vi "novoGoleiroAlinharComATrave.vi"(8 "balls":T1[](array[typedef]), 9 "Robot in":T2, 10 "Goleiro.X_padrao":dbl, 11 "IA State":T7={"our_robots"=[], "enemy_robots"=[], "balls"=[], "geometry"={"field_length"=0, "field_width"=0, "goal_width"=0, "goal_depth"=0, "center_circle_radius"=0, "defense_width"=0, "defense_depth"=0, "free_kick_from_defense_dist"=0, "penalty_spot_from_field_line_dist"=0, "penalty_line_from_spot_dist"=0, "half_moon_depth"=0, "half_moon_width"=0}, "IA Judge"={"stage"="", "command"="", "our_goalie_id"=0.0, "enemy_goalie_id"=0.0, "command enum"=enum."Halt", "Time"=enum."Azul"}, "Received Timestamp"=timestamp(0 s since 1904-01-01), "Events"={"Touch"=FALSE, "id touch"=0.0, "Ball out of \nVision"=FALSE, "Ball inside \nGoalie area"=FALSE, "Robot not responding"=FALSE, "Robots responding status"=[1.0, 1.0, 1.0, 1.0, 1.0, 1.0], "Enemy Ball \nPossession"=FALSE, "Id ini Possession"=0.0, "Ball Possesion"=FALSE, "Id Possesion"=0.0, "Ball at\nour goal side"=FALSE, "Ball at\ntouchline"=FALSE, "Ball at\nenemy goal side"=FALSE}}) -> (3 "Cluster de saída":T2)   [LabVIEW 2018]
uses:
  2019/VSS/Core/AI Input.ctl
  2019/VSS/Core/AI Robot.ctl
  2019/VSS/Intel/Functions Enum.ctl
  2019/VSS/Intel/AttackerStates.ctl
  2019/VSS/Path Planning/RRT/PathDests.ctl
  2019/VSS/Path Planning/RRT/PathDest.ctl
  2019/VSS/Core/AI Ball.ctl
  2019/VSS/Core/Field Size.ctl
  2019/VSS/Core/AI Judge.ctl
  2019/VSS/Intel/Command Enum.ctl
  2019/VSS/Util/Events/Events.ctl
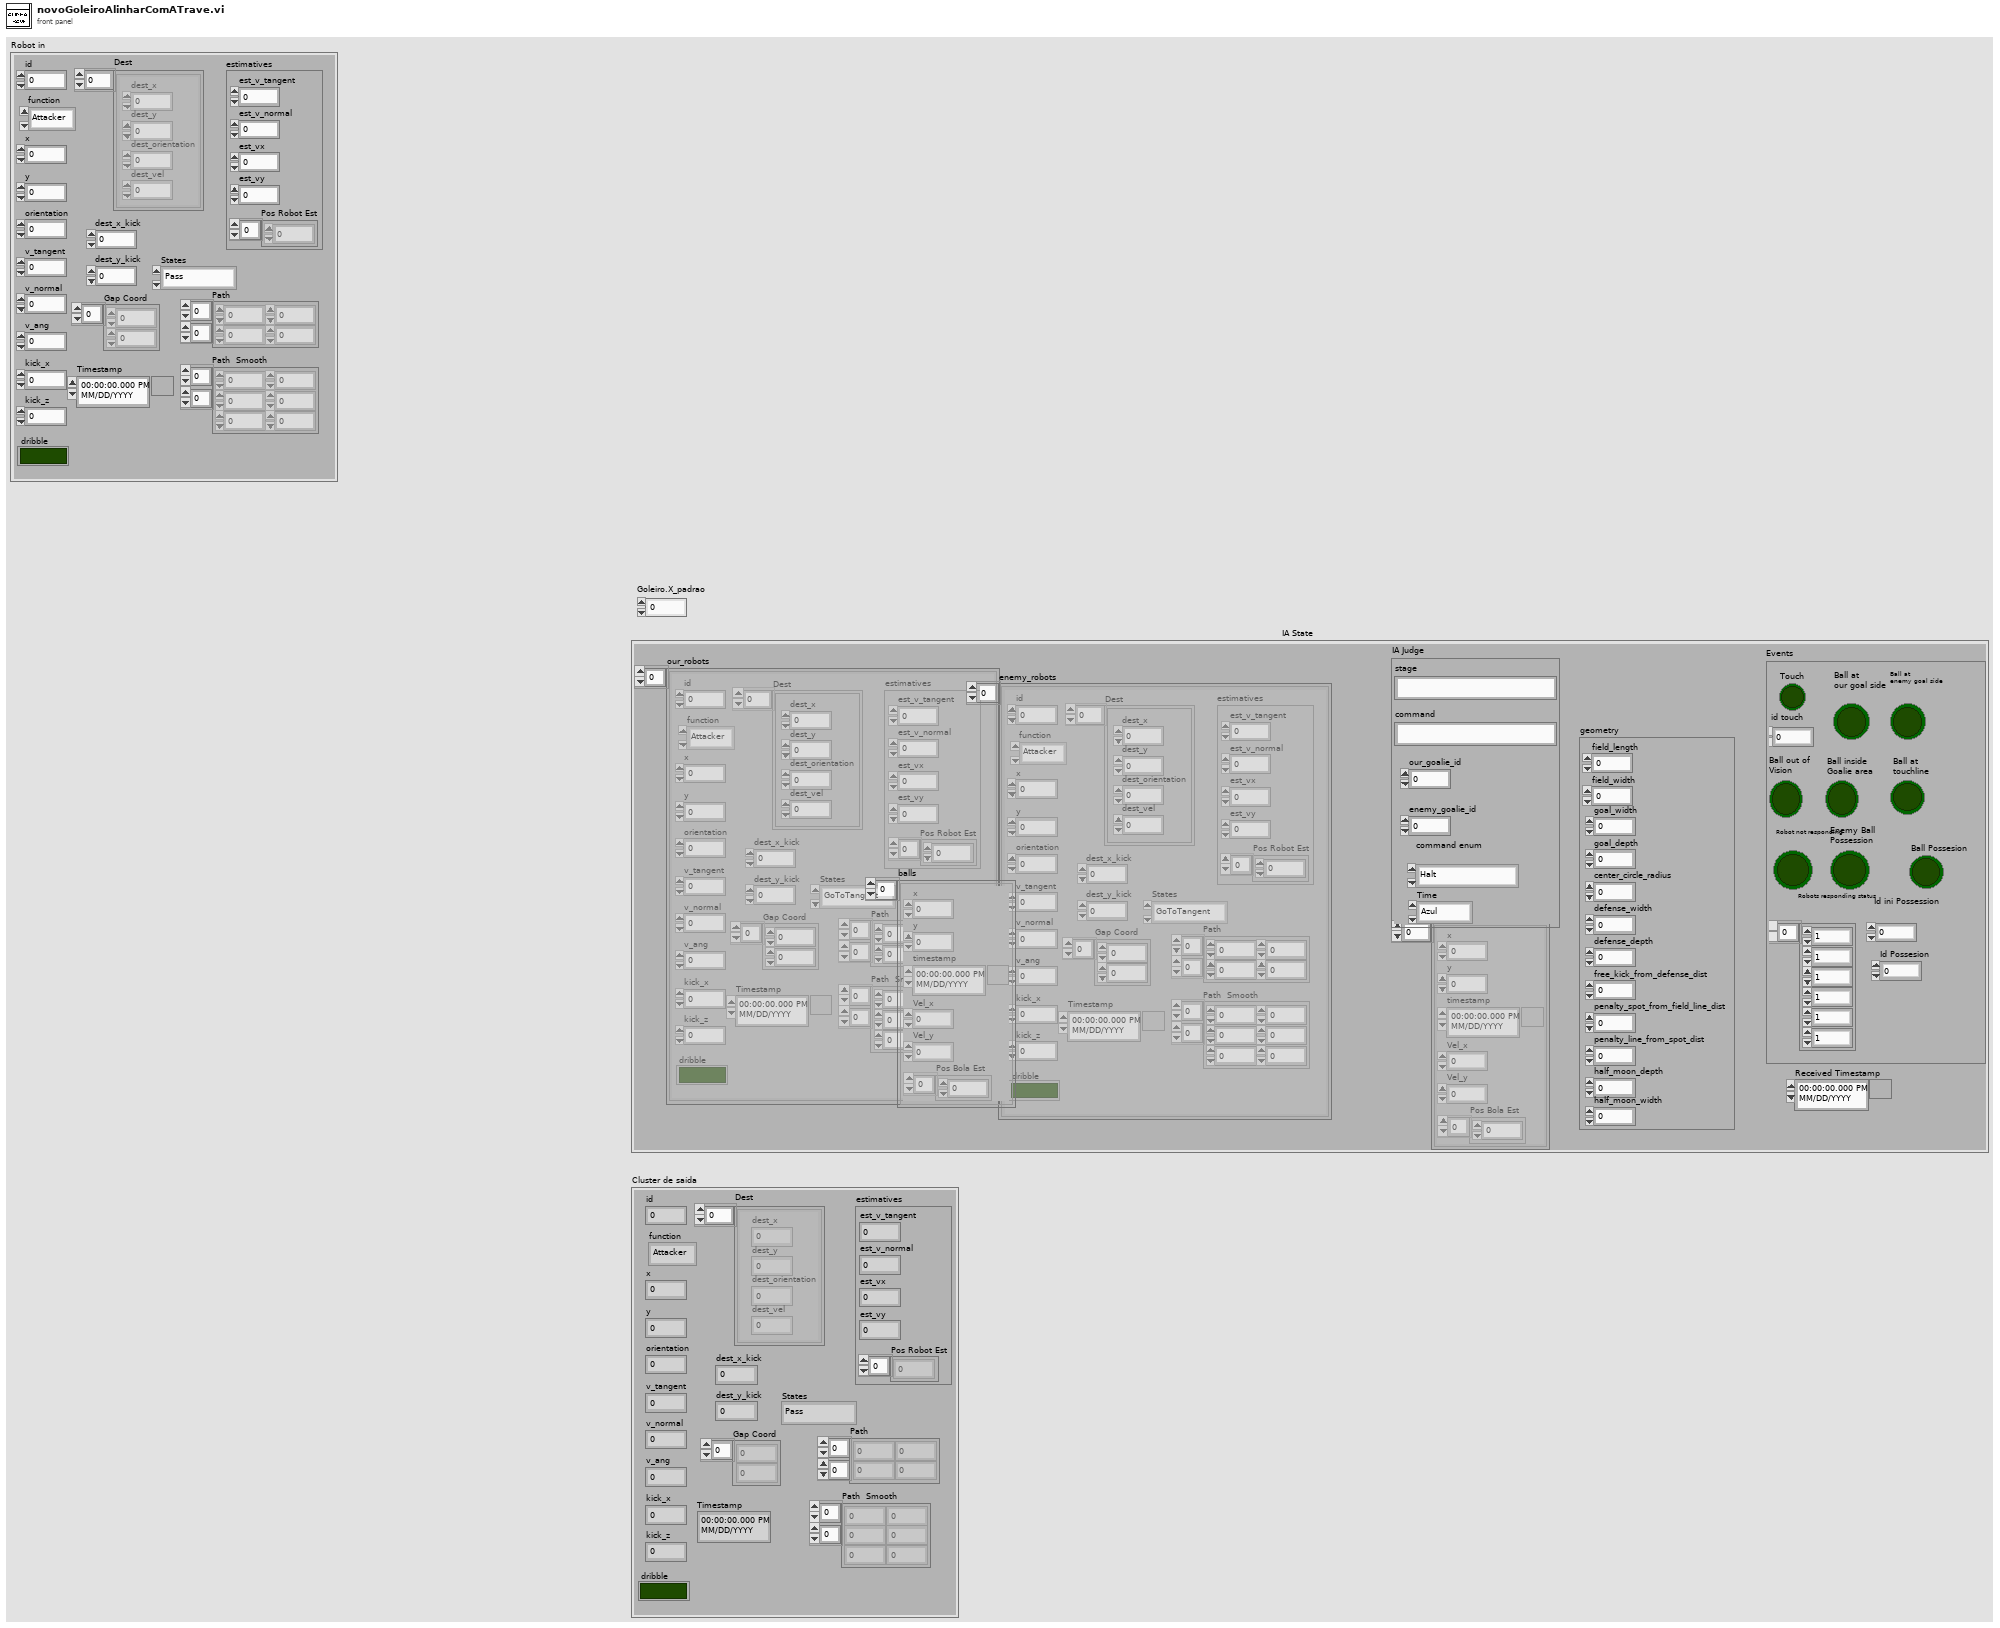
[diagram p1: front panel]
types:
  T1 = typedef "AI Ball.ctl" = cluster{"x":dbl, "y":dbl, "timestamp":timestamp, "Vel_x":dbl, "Vel_y":dbl, "Pos Bola Est":dbl[]}
  T2 = typedef "AI Robot.ctl" = cluster{"id":u32, "function":T3, "x":dbl, "y":dbl, "orientation":dbl, "v_tangent":dbl, "v_normal":dbl, "v_ang":dbl, "kick_x":dbl, "kick_z":dbl, "dribble":bool, "Timestamp":timestamp, "estimatives":cluster{"est_v_tangent":dbl, "est_v_normal":dbl, "est_vx":dbl, "est_vy":dbl, "Pos Robot Est":dbl[]}, "dest_x_kick":dbl, "dest_y_kick":dbl, "Gap Coord":dbl[], "States":T4, "Path ":dbl[][], "Path  Smooth":dbl[][], "Dest":T5}
  T3 = typedef "Functions Enum.ctl" = enum16{"Attacker", "Goalie", "Defender", "Striker", "Goto 0", "Dummy", "Kicker", "ZigZag"}
  T4 = typedef "AttackerStates.ctl" = enum16{"Pass", "GoToTangent", "BallGetting", "GoToKick", "Rotate anti-clockwise", "Rotate Clockwise", ""}
  T5 = typedef "PathDests.ctl" = T6[]
  T6 = typedef "PathDest.ctl" = cluster{"dest_x":dbl, "dest_y":dbl, "dest_orientation":dbl, "dest_vel":dbl}
  T7 = typedef "AI Input.ctl" = cluster{"our_robots":T2[], "enemy_robots":T2[], "balls":T1[], "geometry":T8, "IA Judge":T9, "Received Timestamp":timestamp, "Events":T11}
  T8 = typedef "Field Size.ctl" = cluster{"field_length":u32, "field_width":u32, "goal_width":u32, "goal_depth":u32, "center_circle_radius":u32, "defense_width":u32, "defense_depth":u32, "free_kick_from_defense_dist":u32, "penalty_spot_from_field_line_dist":u32, "penalty_line_from_spot_dist":u32, "half_moon_depth":u32, "half_moon_width":u32}
  T9 = typedef "AI Judge.ctl" = cluster{"stage":string, "command":string, "our_goalie_id":dbl, "enemy_goalie_id":dbl, "command enum":T10, "Time":enum16{"Azul", "Amarelo"}}
  T10 = typedef "Command Enum.ctl" = enum16{"Halt", "Stop", "Force Start", "PKA Normal Start", "Prepare Kickoff Ally", "PKE Normal Start", "Prepare Kickoff Enemy", "Prepare Penalty Ally", "PPA Normal Start", "Prepare Penalty Enemy", "PPE Normal Start", "Ball Placement Enemy Up", "Ball Placement Enemy Down", "Ball Placement Ally Up", "Ball Placement Ally Mid", "Ball Placement Ally Down", "Indirect Free Enemy", "Indirect Free Ally", "Timeout Enemy", "Timeout Ally", "Goal Enemy", "Goal Ally", "Normal Half Time", "Extra Time Break", "Extra Half Time", "None", "Post Game"}
  T11 = typedef "Events.ctl" = cluster{"Touch":bool, "id touch":dbl, "Ball out of \nVision":bool, "Ball inside \nGoalie area":bool, "Robot not responding":bool, "Robots responding status":dbl[], "Enemy Ball \nPossession":bool, "Id ini Possession":dbl, "Ball Possesion":bool, "Id Possesion":dbl, "Ball at\nour goal side":bool, "Ball at\ntouchline":bool, "Ball at\nenemy goal side":bool}
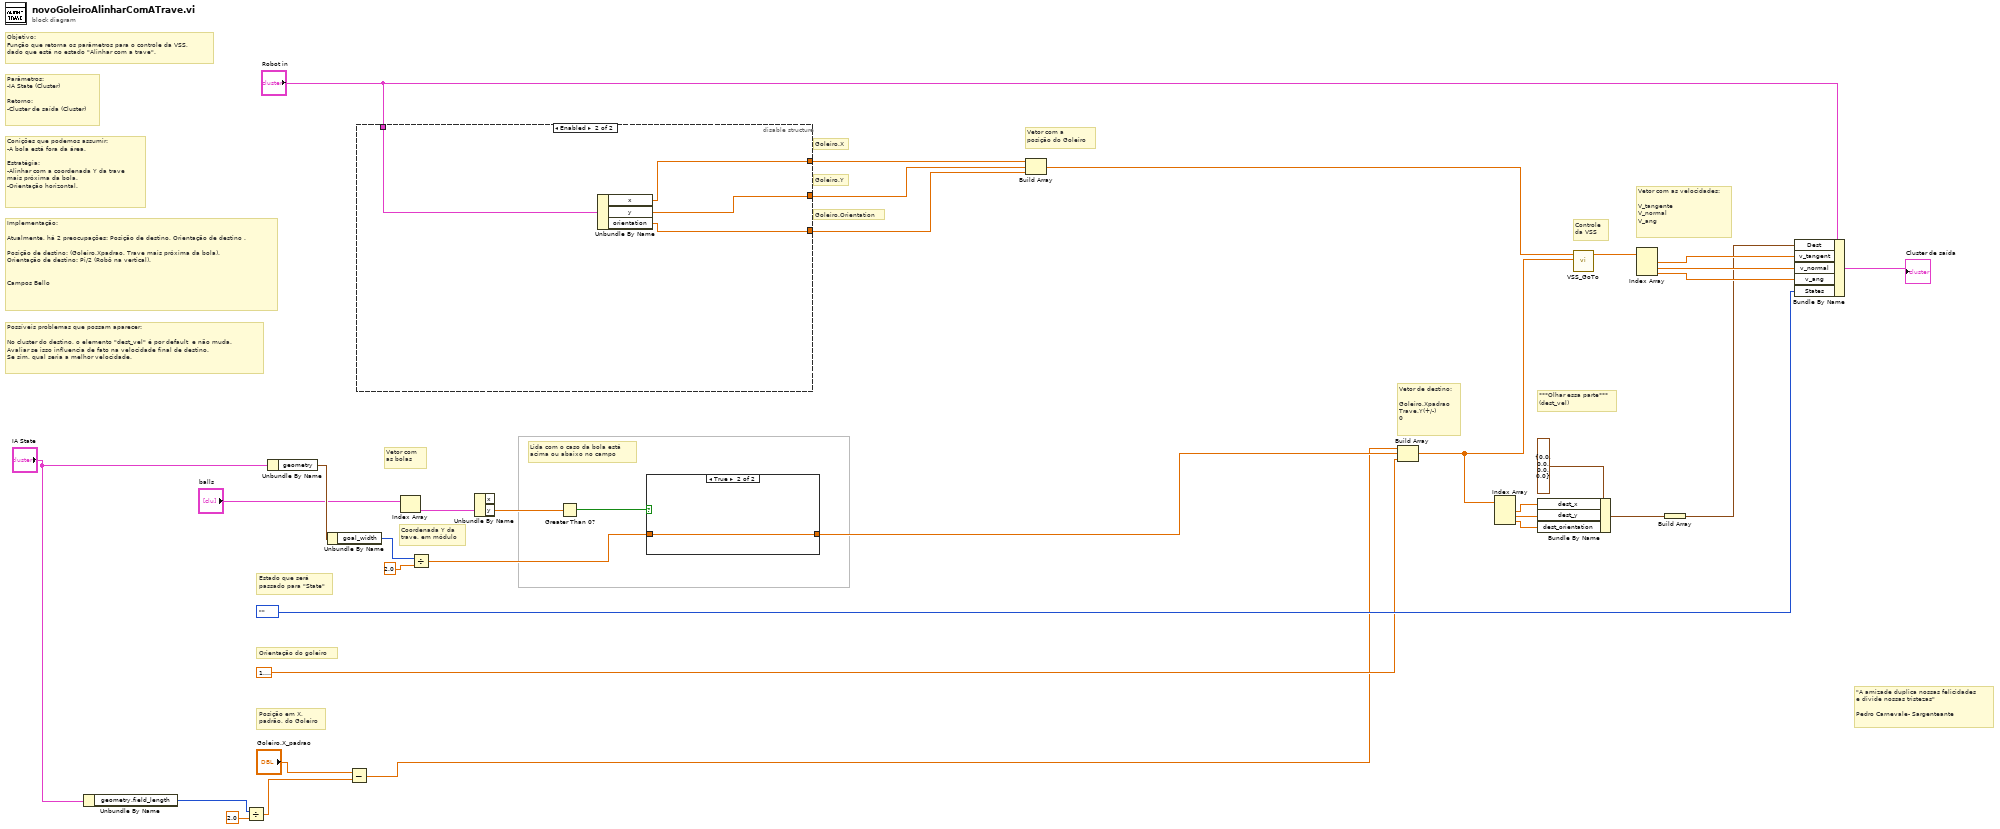
[diagram p0: block diagram]
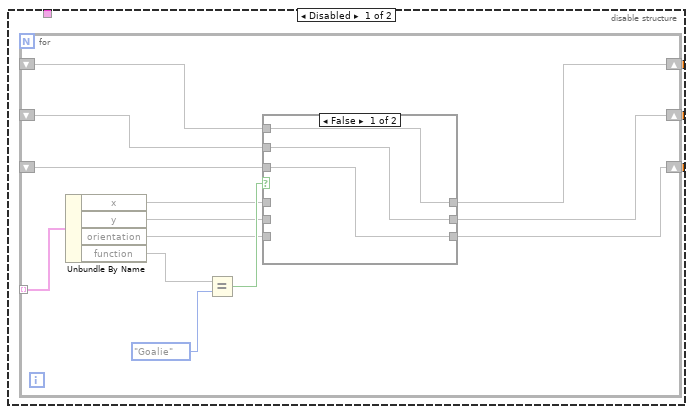
[diagram p2: hidden frame]
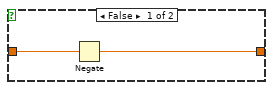
[diagram p4: hidden frame]
diagram:
  # "Lida com o caso da bola está \nacima ou abaixo no campo"
  # "Coordenada Y da\ntrave, em módulo"
  # "\"A amizade duplica nossas felicidades \ne divide nossas tristezas\" \n\nPedro Carnevale- Sargenteante"
  # "Conições que podemos assumir:\n-A bola está fora da área.\n\nEstratégia:\n-Alinhar com a coordenada Y da trave \nmais próxima da bola.\n-Orientação horizontal."
  # "Possíveis problemas que possam aparecer:\n\nNo cluster do destino, o elemento \"dest_vel\" é por default  e não muda. \nAvaliar se isso influencia de fato na velocidade final de destino.\nSe sim, qual seria a melhor velocidade."
  # "Implementação:\n\nAtualmente, há 2 preocupações: Posição de destino, Orientação de destino .\n\nPosição de destino: (Goleiro.Xpadrao, Trave mais próxima da bola).\nOrientação de destino: Pi/2 (Robô na vertical).\n\n\nCampos Bello"
  # "Parâmetros:\n-IA State (Cluster)\n\nRetorno:\n-Cluster de saída (Cluster)"
  # "Objetivo:\nFunção que retorna os parâmetros para o controle da VSS,\ndado que está no estado \"Alinhar com a trave\"."
  # "Posição em X, \npadrão, do Goleiro"
  # "Orientação do goleiro"
  # "Estado que será\npassado para \"State\""
  # "Controle \nda VSS"
  # "***Olhar essa parte***\n(dest_vel)"
  # "Vetor com as velocidades:\n\nV_tangente\nV_normal\nV_ang"
  # "Vetor de destino:\n\nGoleiro.Xpadrao\nTrave.Y(+/-)\n0"
  # "Vetor com \nas bolas"
  # "Vetor com a \nposição do Goleiro"
  # "Goleiro.Orientation"
  # "Goleiro.Y"
  # "Goleiro.X"
  n1 = Unbundle By Name("IA State") -> ("geometry.field_length"=w5:u32)
  n2 = Divide(x=w5, y=2.0) -> (x/y=w4:dbl)
  n3 = Unbundle By Name("IA State") -> ("geometry"=w14:T8)
  n4 = Unbundle By Name(w14) -> ("goal_width"=w12:u32)
  n5 = Subtract(x="Goleiro.X_padrao", y=w4) -> (x-y=w3:dbl)
  n6 = disable-structure shown="Enabled" {
    disable-tunnel: [w38 w60] -> w34
    disable-tunnel: [w37 w58] -> w33
    disable-tunnel: [w36 w59] -> w32
    disable-tunnel: "Robot in" -> [_ w61]
    frame Disabled {
      n7 = for {
        tunnel: [w51] -> w35 mode=indexing
        shift-right: [w45] -> w38
        shift-left: _ -> [w43]
        shift-right: [w44] -> w36
        shift-left: _ -> [w42]
        shift-right: [w40] -> w37
        shift-left: _ -> [w39]
        n8 = Unbundle By Name(w51) -> ("x"=w47, "y"=w46, "orientation"=w41, "function"=w50)
        n9 = Equal?(x=w50, y=Functions_Enum."Goalie" ("function")) -> (x = y?=w48:bool)
        n10 = case shown="False" w48 {
          tunnel: w47 -> [_ w57]
          tunnel: w46 -> [_ w56]
          tunnel: [w54 w57] -> w45
          tunnel: [w53 w56] -> w44
          tunnel: w43 -> [w54 _]
          tunnel: w42 -> [w53 _]
          tunnel: w41 -> [_ w55]
          tunnel: [w52 w55] -> w40
          tunnel: w39 -> [w52 _]
          frame False {
          }
          frame True {
          }
        }
      }
    }
    frame Enabled {
      n11 = Unbundle By Name(w61) -> ("x"=w60:dbl, "y"=w59:dbl, "orientation"=w58:dbl)
    }
  }
  n12 = Index Array(array="balls") -> (element=w31:T1)  [unwired: 1 in]
  n13 = Divide(x=w12, y=2.0 ("x/y")) -> (x/y=w11:dbl)
  n14 = Unbundle By Name(w31) -> ("y"=w16:dbl)  [unwired: 1 out]
  n15 = Greater Than 0?(x=w16) -> (x > 0?=w15:bool)
  n16 = case shown="True" w15 {
    tunnel: w11 -> [w63 w64]
    tunnel: [w62 w64] -> w10
    frame False {
      n17 = Negate(x=w63) -> (-x=w62:dbl)
    }
    frame True {
    }
  }
  n18 = Build Array(w34, w32, w33) -> (w30:dbl[])
  n19 = Build Array(w3, w10, 1.5707963267948966) -> (w24:dbl[])
  n20 = Index Array(array=w24) -> (element #1=w23:dbl, element #2=w22:dbl, element #3=w21:dbl)  [unwired: 3 in]
  n21 = Bundle By Name(cluster=T6 {"dest_x"=0.0, "dest_y"=0.0, "dest_orientation"=0.0, "dest_vel"=0.0} ("element"), "dest_x"=w23, "dest_y"=w22, "dest_orientation"=w21) -> (w20:T6)
  n22 = call "VSS_GoTo.vi"("SetPoint"=w24, "Position"=w30) -> ("Output Vel"=w29:dbl[])  [unwired: 9 in]
  n23 = Index Array(array=w29) -> (element #1=w28:dbl, element #2=w27:dbl, element #3=w26:dbl)  [unwired: 3 in]
  n24 = Build Array(w20) -> (w19:T6[])
  n25 = Bundle By Name(cluster="Robot in", "Dest"=w19, "v_tangent"=w28, "v_normal"=w27, "v_ang"=w26, "States"=AttackerStates."") -> (→"Cluster de saída":T2)
